vi "Lockin Engine.vi"(5 "order":i32=2, 7 "TC (s)":dbl=0.5, 8 "error in (no error)":errorcluster, 10 "Reference In":waveform(dbl)[](array[waveform]), 11 "Signal in":waveform(dbl)[](array[waveform])) -> (0 "error out":errorcluster, 3 "Results (X,Y,R,Theta)":dbl[][](array[numeric]), 4 "filter fC (Hz)":dbl=0.3183098861837907)   [LabVIEW 2016, in "lockin.lvclass"]
uses:
  lockin.lvclass
  <vilib>/Analysis/baseanly.llb/Mean (DBL).vi
  <vilib>/Analysis/NI_AALBase.lvlib
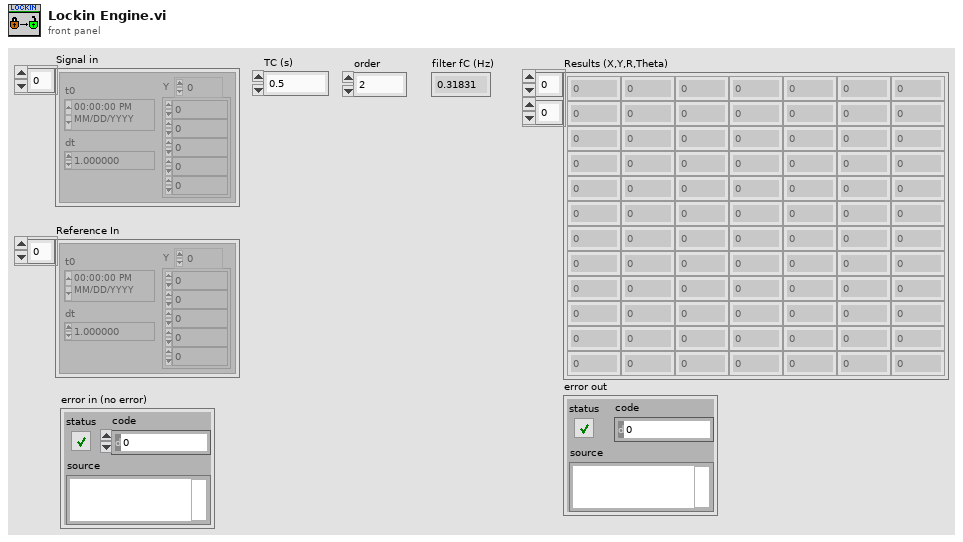
[diagram p1: front panel]
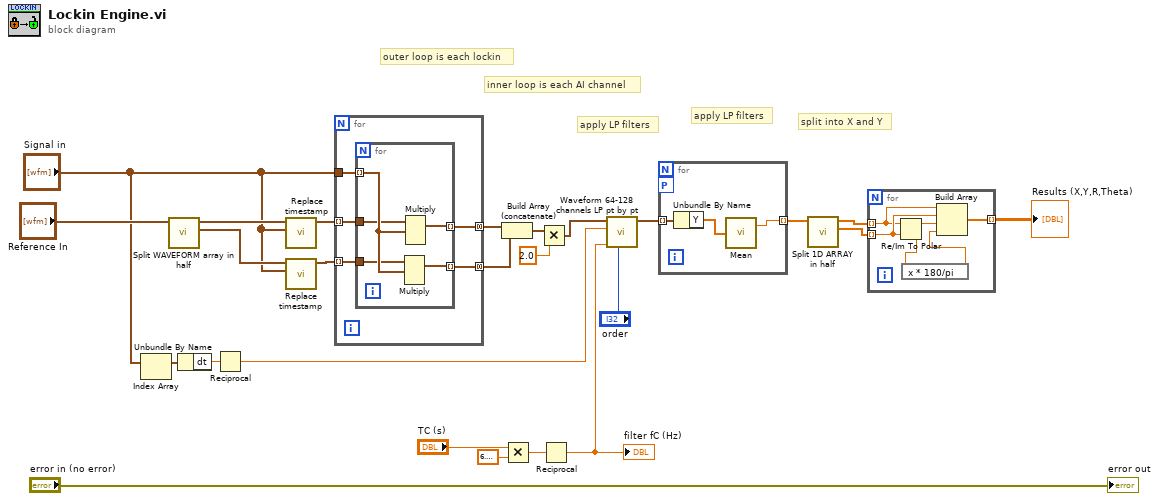
[diagram p0: block diagram]
diagram:
  # "split into X and Y"
  # "apply LP filters"
  # "apply LP filters"
  # "inner loop is each AI channel"
  # "outer loop is each lockin"
  n1 = Index Array(array="Signal in") -> (element=w4:waveform(dbl))  [unwired: 1 in]
  n2 = call "Split WAVEFORM array in half.vi"("AO Array"="Reference In") -> ("Array 2"=w16:waveform(dbl)[], "Array 1"=w15:waveform(dbl)[])  [unwired: 9 in]
  n3 = Unbundle By Name(w4) -> ("dt"=w3:dbl)
  n4 = Reciprocal(x=w3) -> (1/x=w2:dbl)
  n5 = call "Replace timestamp.vi"("Array 2"="Signal in", "Array 1"=w15) -> ("Array Out"=w18:waveform(dbl)[])  [unwired: 9 in]
  n6 = call "Replace timestamp.vi"("Array 2"="Signal in", "Array 1"=w16) -> ("Array Out"=w17:waveform(dbl)[])  [unwired: 9 in]
  n7 = for {
    tunnel: [w30] -> w11 mode=concatenating
    tunnel: [w29] -> w12 mode=concatenating
    tunnel: w17 -> [w28] mode=indexing
    tunnel: w18 -> [w27] mode=indexing
    tunnel: "Signal in" -> [w26]
    n8 = for {
      tunnel: [w35] -> w29 mode=indexing
      tunnel: w28 -> [w31]
      tunnel: w26 -> [w33] mode=indexing
      tunnel: w27 -> [w32]
      tunnel: [w34] -> w30 mode=indexing
      n9 = Multiply(1:w33, 2:w31) -> (0:w35:waveform(dbl))  [unwired: 1 in, 1 out]
      n10 = Multiply(1:w33, 2:w32) -> (0:w34:waveform(dbl))  [unwired: 1 in, 1 out]
    }
  }
  n11 = Build Array (concatenate)(w11, w12) -> (w13:waveform(dbl)[])
  n12 = Multiply(x="TC (s)", y=6.283185307179586) -> (x*y=w9:dbl)
  n13 = Multiply(x=w13, y=2.0) -> (x*y=w25:waveform(dbl)[])
  n14 = Reciprocal(x=w9) -> (1/x=w20:dbl)
  "filter fC (Hz)" <- w20
  n15 = call "Waveform 64-128 channels LP pt by pt.vi"("order"="order", "fl"=w20, "fs"=w2, "Array in"=w25) -> ("Array out"=w21:waveform(dbl)[])  [unwired: 7 in]
  n16 = for {
    tunnel: [w37] -> w22 mode=indexing
    workers-P: _ -> [_]
    tunnel: w21 -> [w36] mode=indexing
    n17 = Unbundle By Name(w36) -> ("Y"=w38:dbl[])
    n18 = call-poly <vilib>:"Mean.vi"("X"=w38) -> ("mean"=w37:dbl)  [unwired: 1 out]
  }
  n19 = call "Split 1D ARRAY in half.vi"("Array in"=w22) -> ("Array out"=w7:dbl[], "Array 3"=w6:dbl[])  [unwired: 9 in]
  n20 = for {
    tunnel: w6 -> [w41] mode=indexing
    tunnel: w7 -> [w43] mode=indexing
    tunnel: [w42] -> w14 mode=indexing
    n21 = Re/Im To Polar(2:w43, 3:w41) -> (0:w40:dbl, 1:w44:dbl)
    n22 = expression code="x * 180/pi"(w40) -> (w39:dbl)
    n23 = Build Array(w41, w43, w44, w39) -> (w42:dbl[])
  }
  "Results (X,Y,R,Theta)" <- w14
  "error out" <- "error in (no error)"
